vi "Tag Throughput.vi"() -> ()   [LabVIEW 2023]
uses:
  <vilib>/Skyline/Tag/Shared/typedefs/DataType.ctl
  <vilib>/Skyline/Tag/Shared/typedefs/Retention Type.ctl
  <vilib>/Skyline/Tag/Wrapper/Wrapper_class/Tag Value Cluster Wrapper.ctl
  <vilib>/Skyline/Configuration/Configuration_class/NI Skyline Configuration.lvclass
  <vilib>/Skyline/Tag/Shared/typedefs/Tag Value Cluster.ctl
  <vilib>/Skyline/Tag/Wrapper/Wrapper_class/Generate Tag Cluster (DBL) 2.vi
  <vilib>/Skyline/Tag/Shared/Serialize Double to String.vi
  <vilib>/Skyline/Utilities/Build Resource Name.vi
  <vilib>/Skyline/Tag/Wrapper/Wrapper_class/Generate Tag Cluster Core 2.vi
  <vilib>/Skyline/Tag/Wrapper/Wrapper_class/Delete Tag (Multiple).vi
  <vilib>/Skyline/Tag/Wrapper/Wrapper_class/NI Skyline Tag.lvclass
  <vilib>/Skyline/Tag/Shared/NI Skyline Tag.lvlib
  <vilib>/Skyline/Tag/Wrapper/Wrapper HTTP_class/NI Skyline Tag HTTP.lvclass
panel:
  out "Init tag loop":i32
  out "error out 2":errorcluster
  out "inner loop":i32
  out "Waveform Chart":u32(graph)
  in  "stop":bool
  out "Write time (mS)":u32
  out "error out":errorcluster
  out "Tag Paths":string[](array[string])
  in  "Updates per tag":i32
  in  "Number of tags":i32
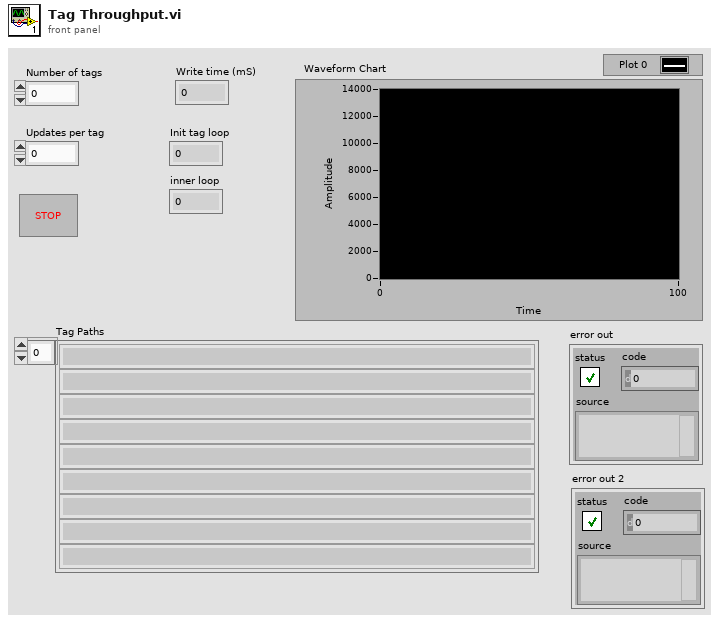
[diagram p1: front panel]
types:
  T1 = typedef "NI Skyline Tag.lvlib/Retention Type.ctl" = enum32{"None", "Duration", "Count", "Permanent"}
  T2 = typedef "NI Skyline Tag.lvlib/DataType.ctl" = enum32{"Double", "I32", "String", "Boolean", "U64", "Timestamp"}
  T3 = typedef "NI Skyline Tag.lvclass/Tag Value Cluster Wrapper.ctl" = cluster{"Configuration":refnum<class "NI Skyline Configuration.lvclass">, "Tag Cluster":T4}
  T4 = typedef "NI Skyline Tag.lvlib/Tag Value Cluster.ctl" = cluster{"Path":string, "Workspace ID":string, "Data Type":T2, "Value":string, "Time Stamp":timestamp}
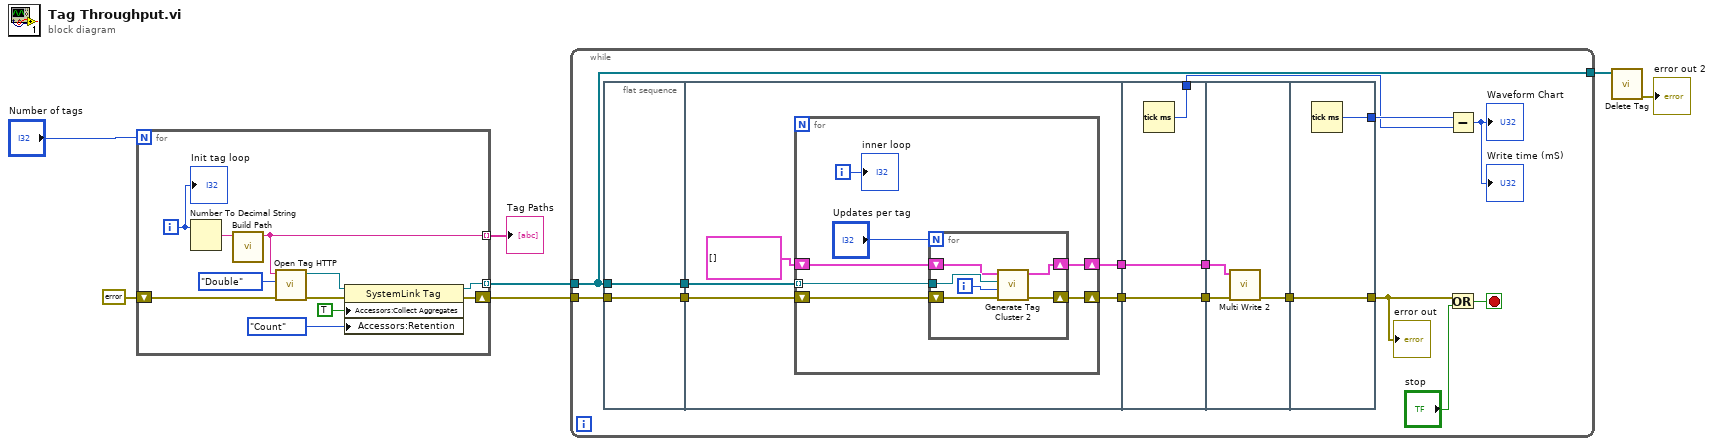
[diagram p0: block diagram]
diagram:
  n1 = for {
    N: "Number of tags" -> [_]
    tunnel: [w17] -> w6 mode=indexing
    tunnel: [w12] -> w5 mode=indexing
    shift-right: [w10] -> w4
    shift-left: errorcluster {"status"=FALSE, "code"=0, "source"=""} ("error out") -> [w15]
    i -> [w14]
    n2 = Number To Decimal String(number=w14) -> (decimal integer string=w18:string)  [unwired: 1 in]
    n3 = call <vilib>:"Build Path.vi"("tag name"=w18) -> ("path"=w17:string)  [unwired: 10 in]
    n4 = call <vilib>:"Open Tag HTTP.vi"("error in (no error)"=w15, "Data Type"=DataType."Double", "path"=w17) -> ("error out"=w11:errorcluster, "tag"=w13:refnum<class "NI Skyline Tag.lvclass">)  [unwired: 7 in]
    n5 = property on="Property Node" class="SystemLink Tag"(reference=w13, error in=w11, "Accessors:Collect Aggregates"=TRUE ("Collect Aggregates"), "Accessors:Retention"=Retention_Type."Count" ("Retention")) -> (reference out=w12:refnum<class "NI Skyline Tag.lvclass">, error out=w10:errorcluster)
    "Init tag loop" <- w14
  }
  "Tag Paths" <- w6
  n6 = while {
    tunnel: w5 -> [w19]
    tunnel: w4 -> [w31]
    tunnel: [w19] -> w2
    stop <- w20 stop-if-true
    n7 = flat-sequence {
      tunnel: w31 -> [w34]
      tunnel: w19 -> [w35]
      tunnel: [w35] -> w33
      tunnel: [w34] -> w32
      tunnel: w33 -> [w40]
      tunnel: w32 -> [w38]
      tunnel: [w37] -> w27
      tunnel: [w36] -> w25
      tunnel: w27 -> [w56]
      tunnel: [w56] -> w26
      tunnel: w25 -> [w55]
      tunnel: [w55] -> w24
      tunnel: [w54] -> w23
      tunnel: [w57] -> w28
      tunnel: w26 -> [w59]
      tunnel: w24 -> [w58]
      tunnel: [w61] -> w22
      tunnel: w28 -> [w61]
      tunnel: [w60] -> w30
      frame #0 {
      }
      frame #1 {
        n8 = for {
          tunnel: w40 -> [w46] mode=indexing
          shift-right: [w44] -> w37
          shift-left: w38 -> [w43]
          shift-right: [w42] -> w36
          shift-left: T3[] [] ("tag clusters in") -> [w47]
          i -> [w41]
          n9 = for {
            N: "Updates per tag" -> [_]
            tunnel: w46 -> [w53]
            shift-right: [w51] -> w44
            shift-left: w43 -> [w50]
            shift-right: [w48] -> w42
            shift-left: w47 -> [w49]
            i -> [w52]
            n10 = call-poly <vilib>:"Generate Tag Cluster 2.vi"("error in (no error)"=w50, "value"=w52, "tag in"=w53, "tag clusters in"=w49) -> ("error out"=w51:errorcluster, "tag clusters out"=w48:T3[])  [unwired: 5 in, 1 out]
          }
          "inner loop" <- w41
        }
      }
      frame #2 {
        n11 = Tick Count (ms)() -> (millisecond timer value=w54:u32)
      }
      frame #3 {
        n12 = call <vilib>:"Multi Write 2.vi"("error in (no error)"=w59, "tag clusters"=w58) -> ("error out"=w57:errorcluster)  [unwired: 9 in]
      }
      frame #4 {
        n13 = Tick Count (ms)() -> (millisecond timer value=w60:u32)
      }
    }
    n14 = Subtract(x=w30, y=w23) -> (x-y=→"Write time (mS)" →"Waveform Chart":u32)
    n15 = Or(x=w22, y="stop") -> (x .or. y?=w20:bool)
    "error out" <- w22
  }
  n16 = call-poly <vilib>:"Delete Tag.vi"("tags"=w2) -> ("error out"=→"error out 2":errorcluster)  [unwired: 10 in]
